vi "Array of Boolean_ASCII String To Data.vi"(8 "error in (no error)":errorcluster, 9 "Default":cluster{"Boolean Array":bool[]}, 11 "Value":string) -> (0 "error out":errorcluster, 3 "Data":cluster{"Boolean Array":bool[]})   [LabVIEW 2020, in "Current Value Table(Rebuild).lvlib"]
doc: "This VI converts data stored on disk as an ascii string into the correct data type. This VI must perform the opposite operation to the DataToASCIIString function."
uses:
  Current Value Table(Rebuild).lvlib
  Errors/Generate Error.vi
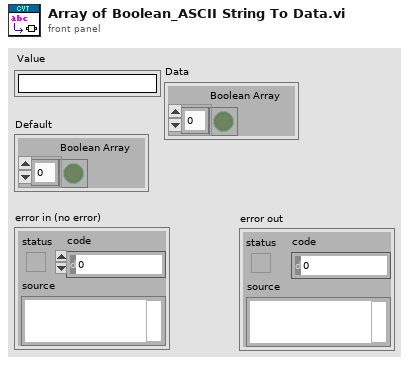
[diagram p1: front panel]
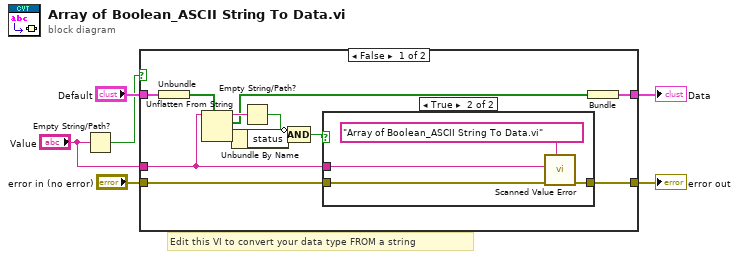
[diagram p0: block diagram]
diagram:
  # "Edit this VI to convert your data type FROM a string"
  n1 = Empty String/Path?(string/path="Value") -> (empty?=w3:bool)
  n2 = case shown="False" w3 {
    tunnel: "Default" -> [w12 w25]
    tunnel: "Value" -> [w10 _]
    tunnel: [w8 w25] -> w1
    tunnel: "error in (no error)" -> [w15 w24]
    tunnel: [w16 w24] -> w5
    frame False {
      n3 = Unbundle(w12) -> ("Boolean Array"=w11:bool[])
      n4 = Unflatten From String(type=w11, binary string=w10) -> (rest of the binary string=w14:string, value=w9:bool[], error out=w13:errorcluster)  [unwired: 3 in]
      n5 = Unbundle By Name(w13) -> ("status"=w7:bool)
      n6 = Empty String/Path?(string/path=w14) -> (empty?=w18:bool)
      n7 = Compound Arithmetic op=AND(invert w18, w7) -> (w17:bool)
      n8 = case shown="True" w17 {
        tunnel: [w19 w23] -> w16
        tunnel: w15 -> [w19 w22]
        tunnel: w10 -> [_ w21]
        frame False {
        }
        frame True {
          n9 = call "Scanned Value Error.vi"("caller name"="Array of Boolean_ASCII String To Data.vi", "error in (no error)"=w22, "Value"=w21) -> ("error out"=w23:errorcluster)  [unwired: 8 in]
        }
      }
      n10 = Bundle("Boolean Array"=w9) -> (w8:cluster{"Boolean Array":bool[]})  [unwired: 1 in]
    }
    frame True {
    }
  }
  "error out" <- w5
  "Data" <- w1
